vi "drawTempLine.vi"(0 "reference":refnum<class "Graphics.lvclass">, 1 "points":T1[](array[typedef]) {"y" format="%.2f"; "x" format="%.2f"}, 2 "lineWidth(1)":dbl=1.0 format="%.2f", 3 "color(if not used=default color)":u32=536870912 format="%.0x", 4 "fill?(F)":bool, 5 "error in (no error)":errorcluster) -> (14 "reference out":refnum<class "Graphics.lvclass">, 16 "new picture":picture, 19 "error out":errorcluster)   [LabVIEW 2020, in "Graphics.lvclass"]
doc: "Draws a temporary line imidielty"
uses:
  <resource>/Framework/Providers/Open_GDS/UML/Graphics_class/Graphics.lvclass
  <resource>/Framework/Providers/Open_GDS/UML/General/Point/Point Point2D.ctl
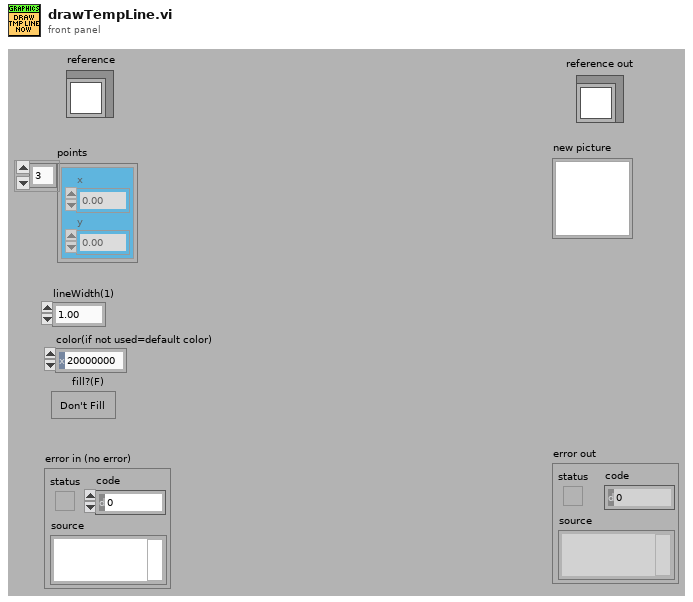
[diagram p1: front panel]
types:
  T1 = typedef "Point Point2D.ctl" = cluster{"x":dbl, "y":dbl}
  T2 = typedef "Graphics.lvclass/ObjectAttributes.ctl" = cluster{"drawColor":u32, "backgroundColor":u32, "font":T3, "fontType":T4, "picture":picture, "stroke":T5, "scaleX":dbl, "scaleY":dbl, "screenRef":refnum<vi>, "offsetX":dbl, "offsetY":dbl}
  T3 = typedef "Graphics.lvclass/FontType.ctl" = cluster{"Font Name:":string, "Size":i16, "Strikeout?":bool, "Italic?":bool, "Underline?":bool, "Outline?":bool, "Shadow?":bool, "Bold?":bool}
  T4 = typedef "Graphics.lvclass/LvFontType.ctl" = enum16{"User-specified Font", "Application Font", "System Font", "Dialog Font"}
  T5 = typedef "Graphics.lvclass/StrokeType.ctl" = enum16{"USE_DEFAULT", "SOLID", "DOTTED"}
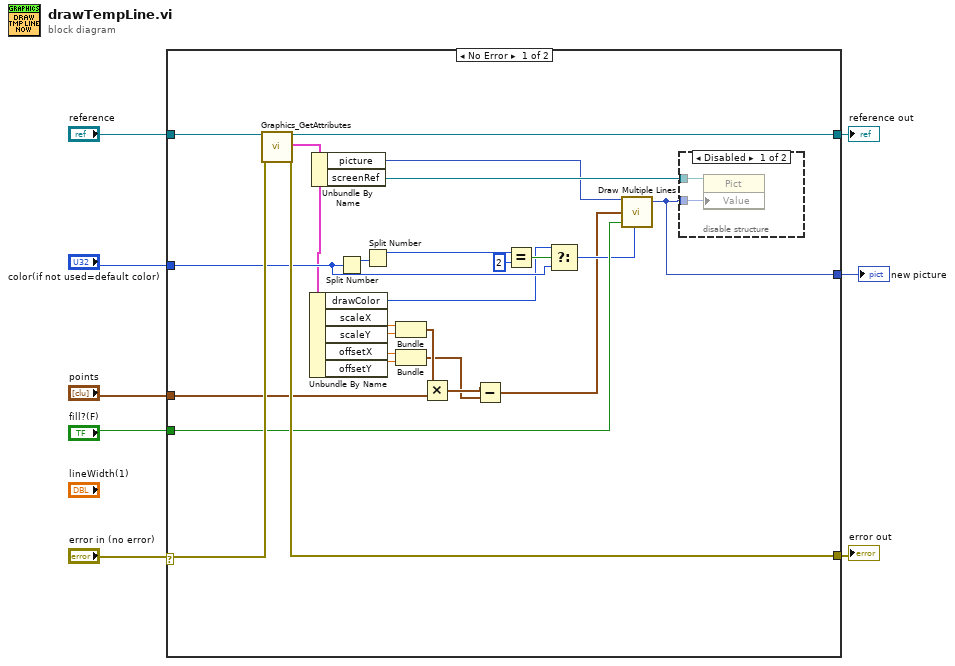
[diagram p0: block diagram]
diagram:
  n1 = case shown="No Error" "error in (no error)" {
    selector: "error in (no error)" -> [w30 w36]
    tunnel: "reference" -> [w33 w37]
    tunnel: [w32 w36] -> w7
    tunnel: [w31 w37] -> w6
    tunnel: "color(if not used=default color)" -> [w29 _]
    tunnel: "points" -> [w28 _]
    tunnel: "fill?(F)" -> [w27 _]
    tunnel: [w9 _] -> w1
    frame No Error {
      n2 = call <resource>:"Graphics_GetAttributes.vi"("reference in"=w33, "error in (no error)"=w30) -> ("reference out"=w31:refnum<class "Graphics.lvclass">, "Data"=w10:T2, "error out"=w32:errorcluster)  [unwired: 1 in, 14 out]
      n3 = Unbundle By Name(w10) -> ("drawColor"=w21:u32, "scaleX"=w19:dbl, "scaleY"=w20:dbl, "offsetX"=w15:dbl, "offsetY"=w14:dbl)
      n4 = Unbundle By Name(w10) -> ("picture"=w18:picture, "screenRef"=w26:refnum<vi>)
      n5 = Split Number(x=w29) -> (hi(x)=w25:u16)  [unwired: 1 out]
      n6 = Split Number(x=w25) -> (hi(x)=w24:u8)  [unwired: 1 out]
      n7 = Bundle("scaleX"=w19, "scaleY"=w20) -> (w16:cluster{"scaleX":dbl, "scaleY":dbl})  [unwired: 1 out]
      n8 = Bundle("offsetX"=w15, "offsetY"=w14) -> (w11:cluster{"offsetX":dbl, "offsetY":dbl})  [unwired: 1 out]
      n9 = Multiply(x=w16, y=w28) -> (x*y=w13:T1[])
      n10 = Subtract(x=w13, y=w11) -> (x-y=w12:T1[])
      n11 = Equal?(x=w24, y=u8 2) -> (x = y?=w22:bool)
      n12 = Select(t=w21, s=w22, f=w29) -> (s? t:f=w17:u32)
      n13 = call <vilib>:"Draw Multiple Lines.vi"("picture"=w18, "line endpoints"=w12, "fill?(F)"=w27, "color(black)"=w17) -> ("new picture"=w9:picture)  [unwired: 1 in, 4 out]
      n14 = disable-structure shown="Disabled" {
        disable-tunnel: w26 -> [w35 _]
        disable-tunnel: w9 -> [w34 _]
        frame Disabled {
          n15 = property class="Pict"(reference=w35, "Value"=w34) -> ()  [unwired: 1 in, 2 out]
        }
        frame Enabled {
        }
      }
    }
    frame Error {
    }
  }
  "reference out" <- w6
  "error out" <- w7
  "new picture" <- w1
